vi "Calibration_MatrixFromTransform.vi"(3 "Transform (Center first)":T1={"Center"={0.0, 0.0}, "Rotate (rad)"=0.0, "MirrorY"=FALSE, "Scale"=1.0}) -> (1 "Linear conversion Matrix":dbl[][](array[numeric]))   [LabVIEW 2011]
panel:
  # "in,1 x LCM = out"
  # "out_i= sum,j (lcm_ij * in _j)"
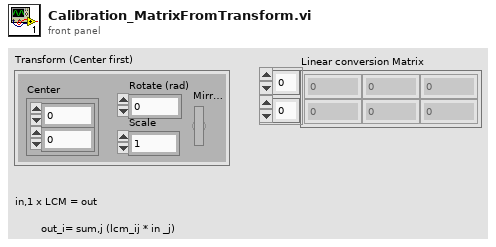
[diagram p1: front panel]
types:
  T1 = cluster{"Center":cluster{dbl, dbl}, "Rotate (rad)":dbl, "MirrorY":bool, "Scale":dbl}
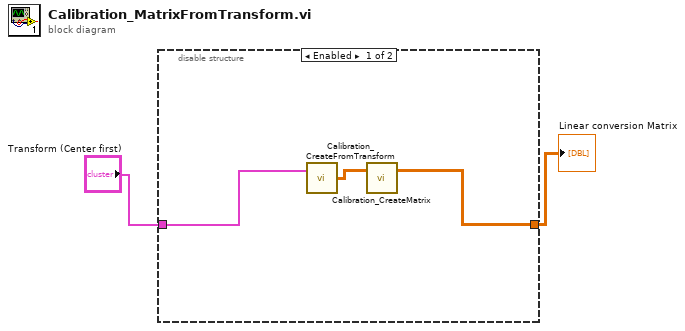
[diagram p0: block diagram]
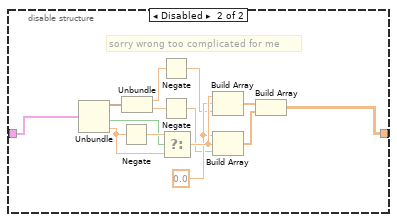
[diagram p2: hidden frame]
diagram:
  n1 = disable-structure shown="Enabled" {
    disable-tunnel: "Transform (Center first)" -> [w5 w7]
    disable-tunnel: [w3 w6] -> w2
    frame Enabled {
      n2 = call "Calibration_CreateFromTransform.vi"("Transform (Center first)"=w5) -> ("CalibrationCoordinates: x,x',y,y'..."=w4:dbl[][])  [unwired: 1 in]
      n3 = call "Calibration_CreateMatrix.vi"("CalibrationCoordinates: x,x',y,y'..."=w4) -> ("Linear conversion Matrix"=w3:dbl[][])  [unwired: 1 in, 1 out]
    }
    frame Disabled {
      w15 = 0.0
      # "sorry wrong too complicated for me"
      n4 = Unbundle(w7) -> ("Center"=w14:cluster{dbl, dbl}, "MirrorY"=w17:bool, "Scale"=w19:dbl)  [unwired: 1 out]
      n5 = Negate(x=w19) -> (-x=w18:dbl)
      n6 = Unbundle(w14) -> (w11:dbl, w10:dbl)
      n7 = Negate(x=w11) -> (-x=w9:dbl)
      n8 = Negate(x=w10) -> (-x=w8:dbl)
      n9 = Select(t=w18, s=w17, f=w19) -> (s? t:f=w16:dbl)
      n10 = Build Array(w16, w15, w9) -> (w13:dbl[])
      n11 = Build Array(w15, w16, w8) -> (w12:dbl[])
      n12 = Build Array(w13, w12) -> (w6:dbl[][])
    }
  }
  "Linear conversion Matrix" <- w2
